vi "Is Attribute a Pointer.vi"(7 "Linked List ID":string, 8 "error in (no error)":errorcluster, 9 "Type":variant, 10 "Attribute Name":string, 11 "ILinked List in":refnum<class "ILinked List.lvclass">) -> (0 "error out":errorcluster, 1 "Pointer ID":string, 2 "Pointer?":bool, 3 "ILinked List out":refnum<class "ILinked List.lvclass">, 4 "Pointer Attribute Name":string)   [LabVIEW 2017, in "Linked Lists.lvlib" / "ILinked List.lvclass"]
uses:
  <vilib>/gpm_packages/@cs/linked-list/Source/Linked List/ILinkedList/ILinked List.lvclass
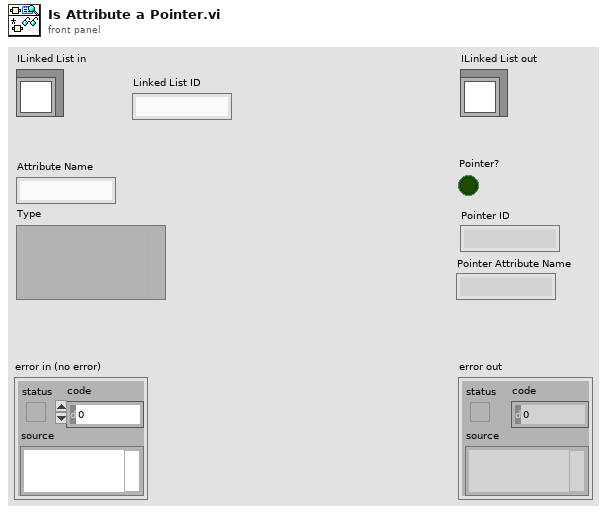
[diagram p1: front panel]
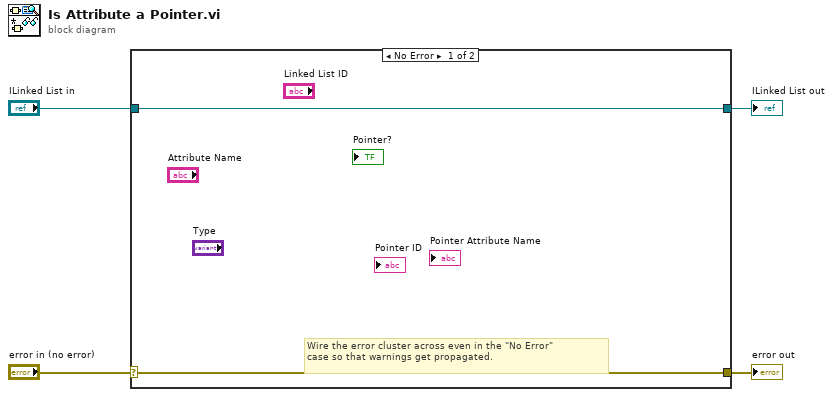
[diagram p0: block diagram]
diagram:
  n1 = case shown="No Error" "error in (no error)" {
    selector: "error in (no error)" -> [w5 w8]
    tunnel: [w5 w8] -> w3
    tunnel: [w6 w7] -> w1
    tunnel: "ILinked List in" -> [w6 w7]
    frame No Error {
      # "Wire the error cluster across even in the \"No Error\"\ncase so that warnings get propagated."
    }
    frame Error {
    }
  }
  "error out" <- w3
  "ILinked List out" <- w1
